vi "DIO64 Set Attribute.vi"(0 "board in":u16 format="%.0x", 5 "attribute id":T2, 7 "attribute value":T1, 9 "value":u32, 11 "error in (no error)":errorcluster) -> (4 "board out":u16 format="%.0x", 15 "error out":errorcluster)   [LabVIEW 2012]
doc: "This VI allows the application to set one of many miscellaneous DIO-64 parameters."
uses:
  DIO64 attribute id.ctl
  DIO64 attribute value.ctl
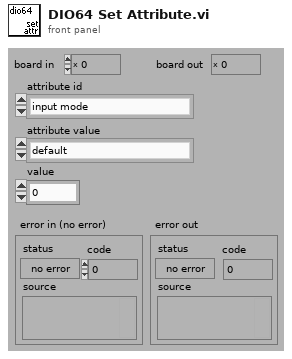
[diagram p1: front panel]
types:
  T1 = typedef "DIO64 attribute value.ctl" = enum16{"default", "long value", "polled", "interrupt", "packet", "demand", "local clock", "external clock", "rtsi/pxi clock", "precision clock", "20MHz", "10MHz", "precision OCXO", "enable", "disable"}
  T2 = typedef "DIO64 attribute id.ctl" = enum16{"input mode", "output mode", "input buffer size", "output buffer size", "major clock source", "input threshold percent", "output threshold percent", "input dma timeout", "rtsi/pxi global enable", "rtsi/pxi clock source", "rtsi clock/pxi trig 7 enable", "external clock enable", "pxi clock enable", "scan clock trig 0 enable", "start trig trig 2 enable", "stop trig trig 3 enable", "daq modulo trig 4 enable", "pxi star enable", "port routing", "staticOutputPorts", "serial number"}
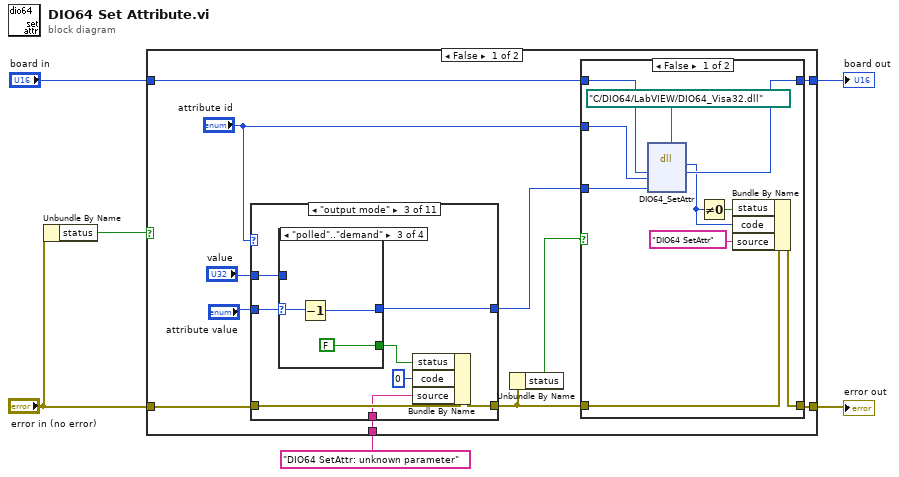
[diagram p0: block diagram]
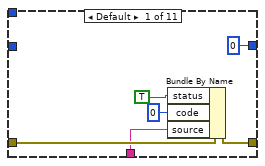
[diagram p3: hidden frame]
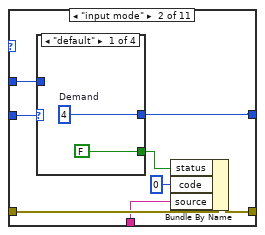
[diagram p4: hidden frame]
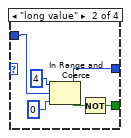
[diagram p5: hidden frame]
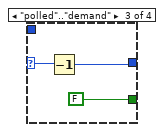
[diagram p6: hidden frame]
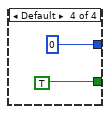
[diagram p7: hidden frame]
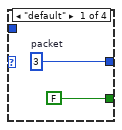
[diagram p8: hidden frame]
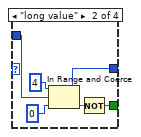
[diagram p9: hidden frame]
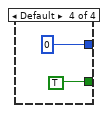
[diagram p10: hidden frame]
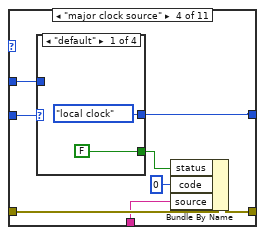
[diagram p11: hidden frame]
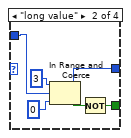
[diagram p12: hidden frame]
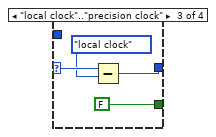
[diagram p13: hidden frame]
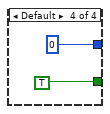
[diagram p14: hidden frame]
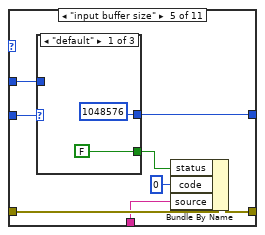
[diagram p15: hidden frame]
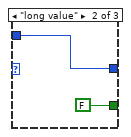
[diagram p16: hidden frame]
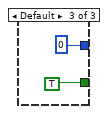
[diagram p17: hidden frame]
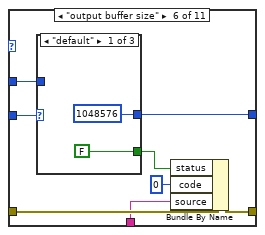
[diagram p18: hidden frame]
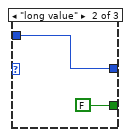
[diagram p19: hidden frame]
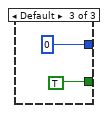
[diagram p20: hidden frame]
diagram:
  n1 = Unbundle By Name("error in (no error)") -> ("status"=w6:bool)
  n2 = case shown="False" w6 {
    tunnel: "error in (no error)" -> [w11 w217]
    tunnel: "board in" -> [w17 w216]
    tunnel: [w16 w216] -> w3
    tunnel: [w15 w217] -> w2
    tunnel: "DIO64 SetAttr: unknown parameter" -> [w8 _]
    frame False {
      n3 = case shown="\"output mode\"" "attribute id" {
        tunnel: "attribute value" -> [_ w43 w64 w85 w107 w121 w135 w153 w171 w189 w205]
        tunnel: "value" -> [_ w42 w63 w84 w106 w120 w134 w152 w170 w188 w204]
        tunnel: w11 -> [w33 w39 w60 w81 w103 w117 w131 w149 w167 w186 w202]
        tunnel: [w34 w38 w59 w80 w102 w116 w130 w148 w166 w185 w201] -> w9
        tunnel: w8 -> [w32 w37 w58 w79 w101 w115 w129 w147 w165 w182 w198]
        tunnel: [u32 0 ("value") w36 w57 w78 w100 w114 w128 w146 w164 w187 w203] -> w7
        frame Default {
          n4 = Bundle By Name(cluster=w33, "status"=TRUE, "code"=0, "source"=w32) -> (w34:errorcluster)
        }
        frame "input mode" {
          n5 = case shown="\"default\"" w43 {
            selector: w43 -> [_ _ w54 _]
            tunnel: w42 -> [_ w49 _ _]
            tunnel: [w45 w48 w53 u32 0] -> w36
            tunnel: [FALSE w47 FALSE TRUE] -> w41
            frame "default" {
              w45 = 4  # Demand
            }
            frame "long value" {
              n6 = In Range and Coerce(upper limit=u32 4, x=w49, lower limit=u32 0 ("upper limit")) -> (coerced(x)=w48:u32, In Range?=w46:bool)
              n7 = Not(x=w46) -> (.not. x?=w47:bool)
            }
            frame "polled".."demand" {
              n8 = Decrement(x=w54) -> (x-1=w53:T1)
            }
            frame Default {
            }
          }
          n9 = Bundle By Name(cluster=w39, "status"=w41, "code"=0, "source"=w37) -> (w38:errorcluster)
        }
        frame "output mode" {
          n10 = case shown="\"polled\"..\"demand\"" w64 {
            selector: w64 -> [_ _ w75 _]
            tunnel: w63 -> [_ w70 _ _]
            tunnel: [w66 w69 w74 u32 0] -> w57
            tunnel: [FALSE w67 FALSE TRUE] -> w62
            frame "default" {
              w66 = 3  # packet
            }
            frame "long value" {
              n11 = In Range and Coerce(upper limit=u32 4, x=w70, lower limit=u32 0 ("upper limit")) -> (coerced(x)=w69:u32, In Range?=w68:bool)
              n12 = Not(x=w68) -> (.not. x?=w67:bool)
            }
            frame "polled".."demand" {
              n13 = Decrement(x=w75) -> (x-1=w74:T1)
            }
            frame Default {
            }
          }
          n14 = Bundle By Name(cluster=w60, "status"=w62, "code"=0, "source"=w58) -> (w59:errorcluster)
        }
        frame "major clock source" {
          n15 = case shown="\"default\"" w85 {
            selector: w85 -> [_ _ w96 _]
            tunnel: w84 -> [_ w91 _ _]
            tunnel: [DIO64_attribute_value."local clock" ("attribute value") w90 w94 u32 0] -> w78
            tunnel: [FALSE w89 FALSE TRUE] -> w83
            frame "default" {
            }
            frame "long value" {
              n16 = In Range and Coerce(upper limit=u32 3, x=w91, lower limit=u32 0 ("upper limit")) -> (coerced(x)=w90:u32, In Range?=w88:bool)
              n17 = Not(x=w88) -> (.not. x?=w89:bool)
            }
            frame "local clock".."precision clock" {
              n18 = Subtract(x=w96, y=DIO64_attribute_value."local clock" ("attribute value")) -> (x-y=w94:u16)
            }
            frame Default {
            }
          }
          n19 = Bundle By Name(cluster=w81, "status"=w83, "code"=0, "source"=w79) -> (w80:errorcluster)
        }
        frame "input buffer size" {
          n20 = case shown="\"default\"" w107 {
            tunnel: w106 -> [_ w111 _]
            tunnel: [u32 1048576 ("value") w111 u32 0 ("value")] -> w100
            tunnel: [FALSE FALSE TRUE] -> w105
            frame "default" {
            }
            frame "long value" {
            }
            frame Default {
            }
          }
          n21 = Bundle By Name(cluster=w103, "status"=w105, "code"=0, "source"=w101) -> (w102:errorcluster)
        }
        frame "output buffer size" {
          n22 = case shown="\"default\"" w121 {
            tunnel: w120 -> [_ w125 _]
            tunnel: [u32 1048576 ("value") w125 u32 0] -> w114
            tunnel: [FALSE FALSE TRUE] -> w119
            frame "default" {
            }
            frame "long value" {
            }
            frame Default {
            }
          }
          n23 = Bundle By Name(cluster=w117, "status"=w119, "code"=0, "source"=w115) -> (w116:errorcluster)
        }
        frame "input threshold percent" {
          n24 = case shown="\"long value\"" w135 {
            tunnel: w134 -> [_ w139 _]
            tunnel: [u32 50 ("value") w138 u32 0] -> w128
            tunnel: [FALSE w140 TRUE] -> w133
            frame "default" {
              # "50%"
            }
            frame "long value" {
              n25 = In Range and Coerce(upper limit=u32 100, x=w139, lower limit=u32 0 ("upper limit")) -> (coerced(x)=w138:u32, In Range?=w143:bool)
              n26 = Not(x=w143) -> (.not. x?=w140:bool)
            }
            frame Default {
            }
          }
          n27 = Bundle By Name(cluster=w131, "status"=w133, "code"=0, "source"=w129) -> (w130:errorcluster)
        }
        frame "output threshold percent" {
          n28 = case shown="\"long value\"" w153 {
            tunnel: w152 -> [_ w157 _]
            tunnel: [u32 50 ("value") w156 u32 0] -> w146
            tunnel: [FALSE w158 TRUE] -> w151
            frame "default" {
              # "50%"
            }
            frame "long value" {
              n29 = In Range and Coerce(upper limit=u32 100, x=w157, lower limit=u32 0 ("upper limit")) -> (coerced(x)=w156:u32, In Range?=w161:bool)
              n30 = Not(x=w161) -> (.not. x?=w158:bool)
            }
            frame Default {
            }
          }
          n31 = Bundle By Name(cluster=w149, "status"=w151, "code"=0, "source"=w147) -> (w148:errorcluster)
        }
        frame "input dma timeout" {
          n32 = case shown="Default" w171 {
            tunnel: w170 -> [_ w175 _]
            tunnel: [u32 100 ("value") w174 u32 0] -> w164
            tunnel: [FALSE w176 TRUE] -> w169
            frame "default" {
              # "100mSec"
            }
            frame "long value" {
              n33 = In Range and Coerce(upper limit=u32 60000, x=w175, lower limit=u32 0 ("upper limit")) -> (coerced(x)=w174:u32, In Range?=w179:bool)
              n34 = Not(x=w179) -> (.not. x?=w176:bool)
            }
            frame Default {
            }
          }
          n35 = Bundle By Name(cluster=w167, "status"=w169, "code"=0, "source"=w165) -> (w166:errorcluster)
        }
        frame "rtsi/pxi global enable" {
          n36 = case shown="\"default\"" w189 {
            tunnel: w188 -> [w190 _ _ _]
            tunnel: [w190 u32 0 ("value") u32 1 ("value") u32 0 ("value")] -> w187
            tunnel: [FALSE ("status") TRUE ("status") FALSE ("status") FALSE ("status")] -> w183
            frame "default" {
            }
            frame Default {
            }
            frame "enable" {
            }
            frame "disable" {
            }
          }
          n37 = Bundle By Name(cluster=w186, "status"=w183, "code"=0, "source"=w182) -> (w185:errorcluster)
        }
        frame "rtsi/pxi clock source" {
          n38 = case shown="\"default\"" w205 {
            tunnel: w204 -> [w206 _ _ _ _]
            tunnel: [w206 u32 0 ("value") u32 0 ("value") u32 1 ("value") u32 2 ("value")] -> w203
            tunnel: [FALSE ("status") TRUE ("status") FALSE ("status") FALSE ("status") FALSE ("status")] -> w199
            frame "default" {
            }
            frame Default {
            }
            frame "20MHz" {
            }
            frame "10MHz" {
            }
            frame "precision OCXO" {
            }
          }
          n39 = Bundle By Name(cluster=w202, "status"=w199, "code"=0, "source"=w198) -> (w201:errorcluster)
        }
      }
      n40 = Unbundle By Name(w9) -> ("status"=w10:bool)
      n41 = case shown="False" w10 {
        tunnel: w17 -> [w27 w29]
        tunnel: [w26 w29] -> w16
        tunnel: [w24 w28] -> w15
        tunnel: w9 -> [w21 w28]
        tunnel: "attribute id" -> [w20 _]
        tunnel: w7 -> [w19 _]
        frame False {
          n42 = dll-call lib="C:/Users/EDM/Desktop/experiment control/subvis/DIO64/DIO64_Visa32.dll" fn="DIO64_SetAttr"(path in=path "C:/DIO64/LabVIEW/DIO64_Visa32.dll", "board"=w27, "attr"=w20, "value"=w19) -> ("return type"=w23:i32, "board"=w26:u16)  [unwired: 3 in, 3 out]
          n43 = Not Equal To 0?(x=w23) -> (x != 0?=w25:bool)
          n44 = Bundle By Name(cluster=w21, "status"=w25, "code"=w23, "source"="DIO64 SetAttr") -> (w24:errorcluster)
        }
        frame True {
        }
      }
    }
    frame True {
    }
  }
  "error out" <- w2
  "board out" <- w3
